vi "CSM - Add Exit State(s) to Queue with Loop Check.vi"(0 "States Out in":string, 5 "Remaining States":string) -> (6 "States Out out":string)   [LabVIEW 2014, in "CSM Loop Support.lvlib"]
uses:
  CSM Loop Support.lvlib
  Communicable State Machine.lvlib
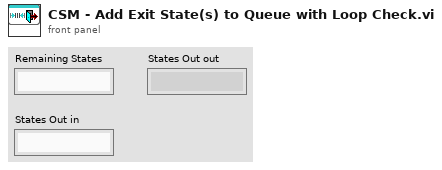
[diagram p1: front panel]
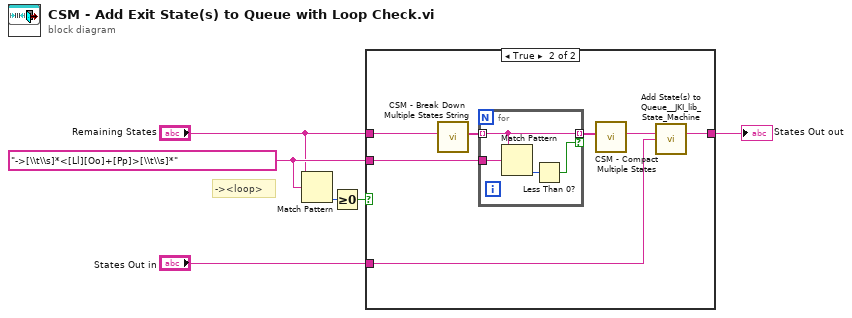
[diagram p0: block diagram]
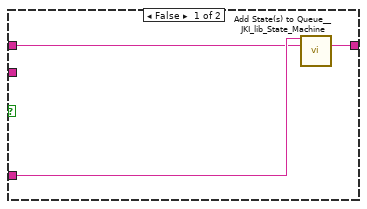
[diagram p2: hidden frame]
diagram:
  w6 = "->[\\t\\s]*<[Ll][Oo]+[Pp]>[\\t\\s]*" ("regular expression")
  # "-><loop>"
  n1 = Match Pattern(string="Remaining States", regular expression=w6) -> (offset past match=w4:i32)  [unwired: 1 in, 3 out]
  n2 = Greater Or Equal To 0?(x=w4) -> (x >= 0?=w5:bool)
  n3 = case shown="True" w5 {
    tunnel: [w9 w13] -> w1
    tunnel: "States Out in" -> [w8 w11]
    tunnel: "Remaining States" -> [w7 w14]
    tunnel: w6 -> [_ w10]
    frame False {
      n4 = call <vilib>:"Add State(s) to Queue__JKI_lib_State_Machine.vi"("State(s) in Front (\"\")"=w8, "State(s) in (\"\")"=w7) -> ("States Out"=w9:string)  [unwired: 13 in]
    }
    frame True {
      n5 = call "CSM - Break Down Multiple States String.vi"("States"=w14) -> ("Multiple States"=w15:string[])  [unwired: 10 in]
      n6 = for {
        tunnel: [w18] -> w16 mode=indexing if=w19
        tunnel: w15 -> [w18] mode=indexing
        tunnel: w10 -> [w17]
        n7 = Match Pattern(string=w18, regular expression=w17) -> (offset past match=w20:i32)  [unwired: 1 in, 3 out]
        n8 = Less Than 0?(x=w20) -> (x < 0?=w19:bool)
      }
      n9 = call "CSM - Compact Multiple States.vi"("Multiple States"=w16) -> ("States"=w12:string)  [unwired: 9 in]
      n10 = call <vilib>:"Add State(s) to Queue__JKI_lib_State_Machine.vi"("State(s) in (\"\")"=w12, "State(s) at Back (\"\")"=w11) -> ("States Out"=w13:string)  [unwired: 13 in]
    }
  }
  "States Out out" <- w1
